vi "Configure Multi Gate Parameters.vi"(7 "Micropulse # In":i32, 8 "error in (no error)":errorcluster, 9 "Multi Gate Inspection":T1={"Gate 1"={"Start (us)"=0.0, "Length (us)"=0.0, "Threshold"=10, "Enabled?"=FALSE, "Max # Peaks"=0, "Hysteresis"=enum."None", "Mode"=enum."1st Peak in Gate", "Inverted?"=FALSE, "Colour "=0}, "Gate 2"={"Start (us)"=0.0, "Length (us)"=0.0, "Threshold"=10, "Enabled?"=FALSE, "Max # Peaks"=0, "Hysteresis"=enum."None", "Mode"=enum."1st Peak in Gate", "Inverted?"=FALSE, "Colour "=0}, "Gate 3"={"Start (us)"=0.0, "Length (us)"=0.0, "Threshold"=10, "Enabled?"=FALSE, "Max # Peaks"=0, "Hysteresis"=enum."None", "Mode"=enum."1st Peak in Gate", "Inverted?"=FALSE, "Colour "=0}, "Gate 4"={"Start (us)"=0.0, "Length (us)"=0.0, "Threshold"=10, "Enabled?"=FALSE, "Max # Peaks"=0, "Hysteresis"=enum."None", "Mode"=enum."1st Peak in Gate", "Inverted?"=FALSE, "Colour "=0}} {"Gate 4"."Max # Peaks" max=64000 step=100; "Gate 4"."Threshold" min=10 max=4095 step=10; "Gate 4"."Length (us)" min=0.0 max=96000.0 step=100.0; "Gate 4"."Start (us)" min=0.0 max=64000.0 step=100.0; "Gate 3"."Max # Peaks" max=64000 step=100; "Gate 3"."Threshold" min=10 max=4095 step=10; "Gate 3"."Length (us)" min=0.0 max=96000.0 step=100.0; "Gate 3"."Start (us)" min=0.0 max=64000.0 step=100.0; "Gate 2"."Max # Peaks" max=64000 step=100; "Gate 2"."Threshold" min=10 max=4095 step=10; "Gate 2"."Length (us)" min=0.0 max=96000.0 step=100.0; "Gate 2"."Start (us)" min=0.0 max=64000.0 step=100.0; "Gate 1"."Max # Peaks" max=64000 step=100; "Gate 1"."Threshold" min=10 max=4095 step=10; "Gate 1"."Length (us)" min=0.0 max=96000.0 step=100.0; "Gate 1"."Start (us)" min=0.0 max=64000.0 step=100.0}, 11 "Test Number":u32) -> (0 "error out":errorcluster, 3 "Test Number out":u32, 5 "Micropulse # Out":i32)   [LabVIEW 2026, in "MicroPulse_Driver.lvlib"]
uses:
  MicroPulse_Driver.lvlib
  Data/Datatypes/MP - multi-gate inspection.ctl
  Data/Datatypes/MP - multigate inspection gate parameters.ctl
  Data/Datatypes/MP - hysteresis level.ctl
  Data/Datatypes/MP - multigate mode.ctl
  <instrlib>/Micropulse/Micropulse.lvlib
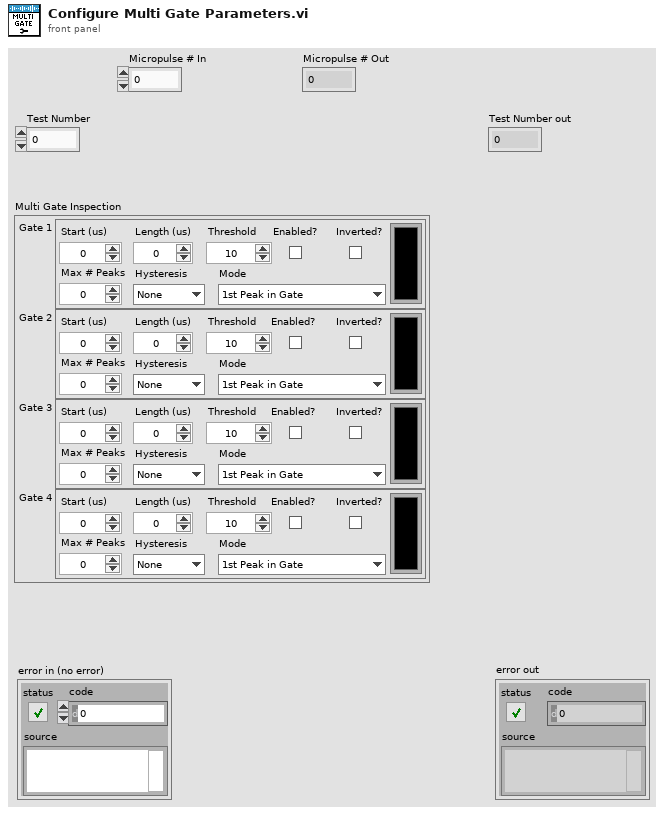
[diagram p1: front panel]
types:
  T1 = typedef "Micropulse.lvlib/MP - multi-gate inspection.ctl" = cluster{"Gate 1":T2, "Gate 2":T2, "Gate 3":T2, "Gate 4":T2}
  T2 = typedef "Micropulse.lvlib/MP - multigate inspection gate parameters.ctl" = cluster{"Start (us)":dbl, "Length (us)":dbl, "Threshold":u16, "Enabled?":bool, "Max # Peaks":u16, "Hysteresis":T3, "Mode":T4, "Inverted?":bool, "Colour ":u32}
  T3 = typedef "Micropulse.lvlib/MP - hysteresis level.ctl" = enum16{"None", "3dB", "6dB", "9dB", "12dB"}
  T4 = typedef "Micropulse.lvlib/MP - multigate mode.ctl" = enum16{"1st Peak in Gate", "Largest Peak In Gate", "All Peaks In Gate", "1st Threshold Crossing"}
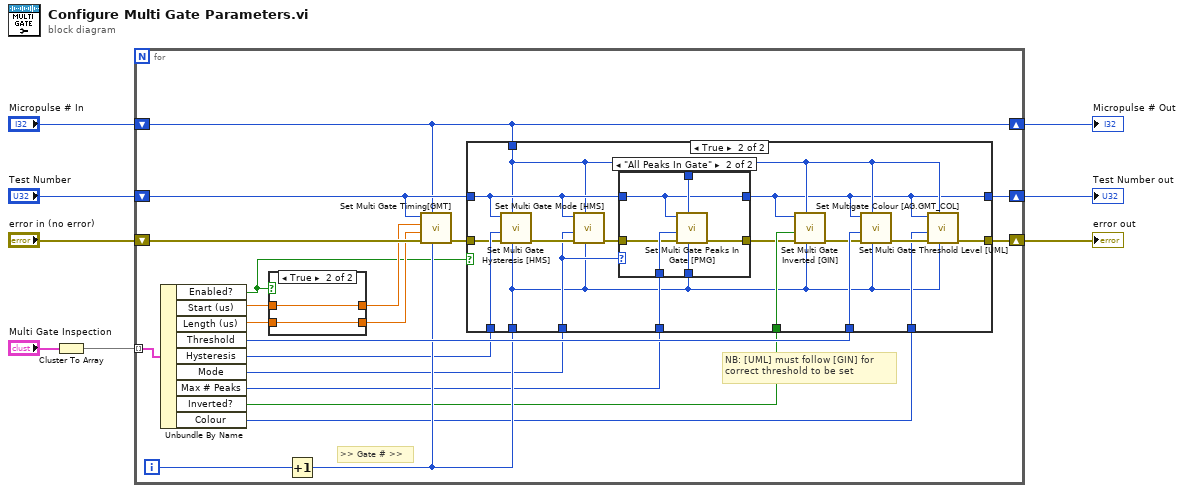
[diagram p0: block diagram]
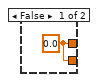
[diagram p4: hidden frame]
diagram:
  n1 = Cluster To Array(cluster="Multi Gate Inspection") -> (array=w4:T2[])
  n2 = for {
    tunnel: w4 -> [w26] mode=indexing
    shift-right: [w12] -> w8
    shift-left: "Micropulse # In" -> [w12]
    shift-right: [w28] -> w6
    shift-left: "error in (no error)" -> [w25]
    shift-right: [w16] -> w1
    shift-left: "Test Number" -> [w27]
    i -> [w18]
    # "NB: [UML] must follow [GIN] for\ncorrect threshold to be set"
    # ">> Gate # >>"
    n3 = Unbundle By Name(w26) -> ("Enabled?"=w15:bool, "Start (us)"=w22:dbl, "Length (us)"=w21:dbl, "Threshold"=w23:u16, "Hysteresis"=w13:T3, "Mode"=w11:T4, "Max # Peaks"=w14:u16, "Inverted?"=w10:bool, "Colour"=w9:u32)
    n4 = case shown="True" w15 {
      tunnel: w22 -> [_ w58]
      tunnel: w21 -> [_ w57]
      tunnel: [w56 w58] -> w20
      tunnel: [w56 w57] -> w19
      frame False {
        w56 = 0.0 ("Start (us)")
      }
      frame True {
      }
    }
    n5 = Increment(x=w18) -> (x+1=w17:i32)
    n6 = call "Set Multi Gate Timing[GMT].vi"("Gate Number"=w17, "Micropulse # In"=w12, "error in (no error)"=w25, "Gate Length (us)"=w19, "Gate Start (us)"=w20, "Test Number"=w27) -> ("error out"=w24:errorcluster)  [unwired: 4 in, 1 out]
    n7 = case shown="True" w15 {
      tunnel: [w30 w35] -> w28
      tunnel: w23 -> [_ w47]
      tunnel: w27 -> [w29 w41]
      tunnel: w24 -> [w30 w37]
      tunnel: w17 -> [_ w31]
      tunnel: [w29 w33] -> w16
      tunnel: w14 -> [_ w46]
      tunnel: w13 -> [_ w45]
      tunnel: w12 -> [_ w34]
      tunnel: w11 -> [_ w42]
      tunnel: w10 -> [_ w40]
      tunnel: w9 -> [_ w32]
      frame False {
      }
      frame True {
        n8 = call "Set Multi Gate Hysteresis [HMS].vi"("Gate Number"=w31, "Micropulse # In"=w34, "error in (no error)"=w37, "Hysteresis"=w45, "Test Number"=w41) -> ("error out"=w44:errorcluster)  [unwired: 5 in, 1 out]
        n9 = call "Set Multi Gate Mode [HMS].vi"("Gate Number"=w31, "Micropulse # In"=w34, "error in (no error)"=w44, "Mode"=w42, "Test Number"=w41) -> ("error out"=w43:errorcluster)  [unwired: 5 in, 1 out]
        n10 = case shown="\"All Peaks In Gate\"" w42 {
          tunnel: [w48 w55] -> w39
          tunnel: w34 -> [_ w54]
          tunnel: w46 -> [_ w53]
          tunnel: w31 -> [_ w52]
          tunnel: w43 -> [w48 w51]
          tunnel: w41 -> [w49 w50]
          tunnel: [w49 w50] -> w33
          frame Default {
          }
          frame "All Peaks In Gate" {
            n11 = call "Set Multi Gate Peaks In Gate [PMG].vi"("Gate Number"=w52, "Micropulse # In"=w54, "error in (no error)"=w51, "# Peaks In Gate"=w53, "Test Number"=w50) -> ("error out"=w55:errorcluster)  [unwired: 5 in, 1 out]
          }
        }
        n12 = call "Set Multi Gate Inverted [GIN].vi"("Gate Number"=w31, "Micropulse # In"=w34, "error in (no error)"=w39, "Inverted?"=w40, "Test Number"=w33) -> ("error out"=w38:errorcluster)  [unwired: 5 in, 1 out]
        n13 = call "Set Multi Gate Threshold Level [UML].vi"("Gate Number"=w31, "Micropulse # In"=w34, "error in (no error)"=w38, "Threshold"=w47, "Test Number"=w33) -> ("error out"=w36:errorcluster)  [unwired: 5 in, 1 out]
        n14 = call "Set Multigate Colour [AG.GMT_COL].vi"("Gate Number"=w31, "Micropulse # In"=w34, "error in (no error)"=w36, "Colour"=w32, "Test Number"=w33) -> ("error out"=w35:errorcluster)  [unwired: 5 in, 1 out]
      }
    }
  }
  "Micropulse # Out" <- w8
  "error out" <- w6
  "Test Number out" <- w1
